vi "Periodic Tasks.vi"(8 "error in":errorcluster) -> ()   [LabVIEW 2014]
doc: "This VI runs in parallel to other tasks. It can contain as many user-defined periodic loops as you need. These can carry out PID or other sorts of timed response."
uses:
  <vilib>/Rock Robotics/WPI/Joystick/WPI_JoystickGetSetRefNum.vi
  <vilib>/Rock Robotics/WPI/RobotDrive/WPI_RobotDriveGetSetRefNum.vi
  Modules 2015/Desired Arm Position.vi
  Robot Global Data.vi
  <vilib>/Rock Robotics/Network Tables/SD Write Number.vi
panel:
  out "Voltage":dbl
  out "desired position":T1(graph)={"Desired Back Arm Position"=13.083464566929848, "Back Arm Distance (inches)"=14.0325}
  out "voltage 2":dbl
  out "Desired Back Arm Position":dbl
  in  "kd 2":dbl=0.01 format="%#_13g"
  in  "kp 2":dbl=0.15 format="%#_13g"
  out "voltage":dbl
  out "Desired Front Arm Position":dbl
  in  "kd":dbl=0.02 format="%#_13g"
  in  "kp":dbl=0.1 format="%#_13g"
  out "Front Arm Distance":dbl
  out "Back Arm Distance":dbl
  out "Angle":dbl
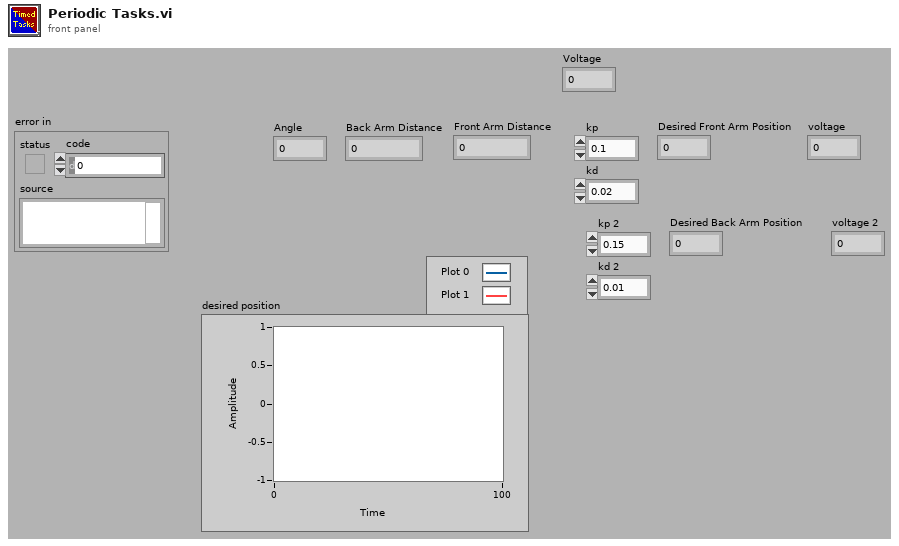
[diagram p1: front panel]
types:
  T1 = cluster{"Desired Back Arm Position":dbl, "Back Arm Distance (inches)":dbl}
  T2 = typedef "WPI_AnalogChannelDevRef.ctl" = cluster{"DevStatus":errorcluster, "Controller":T3, "Analog Channel":T4}
  T3 = typedef "FPGA_TypedefAnalogModule.ctl" = enum16{"Controller 1"}
  T4 = typedef "FPGA_AIChannel.ctl" = enum8{"AI 0", "AI 1", "AI 2", "AI 3", "AI MXP 0", "AI MXP 1", "AI MXP 2", "AI MXP 3", "Invalid"}
  T5 = typedef "WPI_DigitalInputDevRef.ctl" = cluster{"DevStatus":errorcluster, "DIO Channel":T6, "Controller":T7}
  T6 = typedef "FPGA_DIOChannel.ctl" = enum8{"DIO 0", "DIO 1", "DIO 2", "DIO 3", "DIO 4", "DIO 5", "DIO 6", "DIO 7", "DIO 8", "DIO 9", "DIO MXP 0", "DIO MXP 1", "DIO MXP 2", "DIO MXP 3", "DIO MXP 4", "DIO MXP 5", "DIO MXP 6", "DIO MXP 7", "DIO MXP 8", "DIO MXP 9", "DIO MXP 10", "DIO MXP 11", "DIO MXP 12", "DIO MXP 13", "DIO MXP 14", "DIO MXP 15", "Invalid"}
  T7 = typedef "FPGA_TypedefDigitalModule.ctl" = enum16{"Controller 1"}
  T8 = typedef "WPI_JoystickDevRef.ctl" = cluster{"Device":T9}
  T9 = typedef "WPI_JoystickDeviceEnum.ctl" = enum16{"USB 0", "USB 1", "USB 2", "USB 3", "USB 4", "USB 5"}
  T10 = typedef "WPI_RobotDriveDevRef.ctl" = cluster{"DevStatus":errorcluster, "Motors[]":T11[], "Square Inputs":bool, "Max Output":dbl}
  T11 = typedef "WPI_MotorControlDeviceRef.ctl" = cluster{"DeviceStatus":errorcluster, "Type":T12, "PWM":cluster{"Controller":T7, "PWM Channel":T13, "DeadBand":T14}, "CAN":cluster{"Device Number":u8, "Control Mode":T15, "Semaphore":T16, "Max Vout":dbl, "TalonSRX Control Mode":T17}, "Invert":bool, "TransformRef":T18, "InvTransformRef":T18}
  T12 = typedef "WPI_MotorControlType.ctl" = enum16{"PWM", "CAN", "CANTalonSRX"}
  T13 = typedef "FPGA_DIOPWMChannel.ctl" = enum8{"PWM 0", "PWM 1", "PWM 2", "PWM 3", "PWM 4", "PWM 5", "PWM 6", "PWM 7", "PWM 8", "PWM 9", "PWM MXP 0", "PWM MXP 1", "PWM MXP 2", "PWM MXP 3", "PWM MXP 4", "PWM MXP 5", "PWM MXP 6", "PWM MXP 7", "PWM MXP 8", "PWM MXP 9", "Invalid"}
  T14 = typedef "WPI_PWMDeadband.ctl" = cluster{"Name":string, "maxPositivePwm":i32, "minPositivePwm":i32, "centerPwm":i32, "maxNegativePwm":i32, "minNegativePwm":i32, "angularRange":u16}
  T15 = typedef "WPI_CANJaguar_ControlMode.ctl" = enum8{"Percent VBus", "Current", "Speed", "Position", "Voltage"}
  T16 = typedef "Semaphore RefNum" = refnum<k1>
  T17 = typedef "WPI_CANTalonSRX_APIControlMode.ctl" = enum8{"Percent VBus", "Speed", "Position", "Slave", "Unchanged / Invalid"}
  T18 = typedef "WPI_PWMTransform_ConPane.ctl" = refnum<vi>
  T19 = typedef "WPI_EncoderDevRef.ctl" = cluster{"DevStatus":errorcluster, "EncoderIndex":T20, "CounterIndex":T21, "DistancePerCount":dbl, "Decoding Type":T22}
  T20 = typedef "FPGA_EncoderIdx.ctl" = enum8{"Enc 0", "Enc 1", "Enc 2", "Enc 3", "Enc 4", "Enc 5", "Enc 6", "Enc 7", "Invalid"}
  T21 = typedef "FPGA_CounterCtrSystemIndex.ctl" = enum8{"Ctr 0", "Ctr 1", "Ctr 2", "Ctr 3", "Ctr 4", "Ctr 5", "Ctr 6", "Ctr 7", "Invalid"}
  T22 = typedef "WPI_EncoderType.ctl" = enum16{"1x", "2x", "4x"}
  T23 = cluster{"JoystickDevRef":T8, "RobotDriveDevRef":T10}
  T24 = typedef "WPI_GyroDevRef.ctl" = cluster{"DevStatus":errorcluster, "Analog Module":T3, "Analog Channel":T4, "Offset":dbl, "Gain (VoltsPerDegree/Second)":dbl}
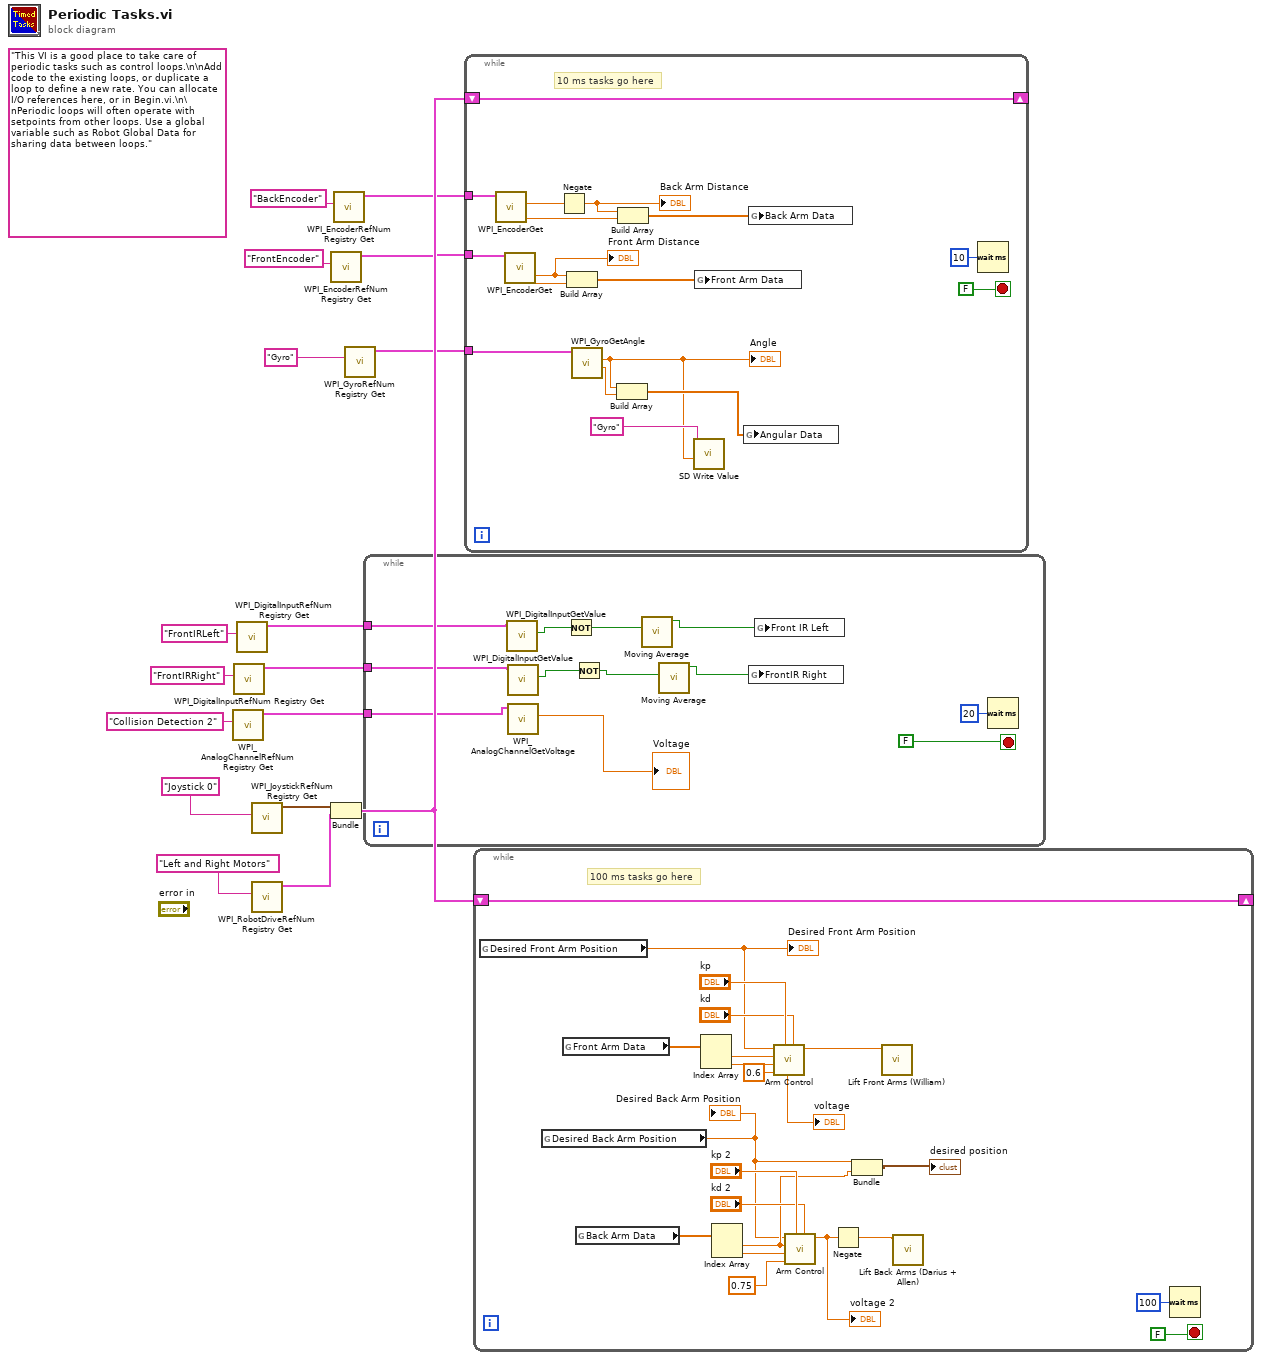
[diagram p0: block diagram]
diagram:
  (unwired) "This VI is a good place to take care of periodic tasks such as control loops.\n\nAdd code to the existing loops, or duplicate a loop to define a new rate. You can allocate I/O references here, or in Begin.vi.\n\nPeriodic loops will often operate with setpoints from other loops. Use a global variable such as Robot Global Data for sharing data between loops."
  n1 = call <vilib>:"WPI_AnalogChannelRefNum Registry Get.vi"("refnum name"="Collision Detection 2") -> ("AIDeviceRef"=w2:T2)  [unwired: 9 in, 1 out]
  n2 = call <vilib>:"WPI_DigitalInputRefNum Registry Get.vi"("refnum name"="FrontIRRight") -> ("DigitalInputDevRef"=w3:T5)  [unwired: 9 in, 1 out]
  n3 = call <vilib>:"WPI_DigitalInputRefNum Registry Get.vi"("refnum name"="FrontIRLeft") -> ("DigitalInputDevRef"=w4:T5)  [unwired: 9 in, 1 out]
  n4 = call <vilib>:"WPI_JoystickRefNum Registry Get.vi"("refnum name"="Joystick 0") -> ("JoystickDevRef"=w15:T8)  [unwired: 1 in, 9 out]
  n5 = call <vilib>:"WPI_RobotDriveRefNum Registry Get.vi"("refnum name"="Left and Right Motors") -> ("RobotDriveDevRef"=w14:T10)  [unwired: 1 in, 9 out]
  n6 = call <vilib>:"WPI_EncoderRefNum Registry Get.vi"("refnum name"="FrontEncoder") -> ("EncoderDevRef"=w5:T19)  [unwired: 9 in, 1 out]
  n7 = Bundle("JoystickDevRef"=w15, "RobotDriveDevRef"=w14) -> (w13:T23)  [unwired: 1 out]
  n8 = call <vilib>:"WPI_EncoderRefNum Registry Get.vi"("refnum name"="BackEncoder") -> ("EncoderDevRef"=w9:T19)  [unwired: 9 in, 1 out]
  n9 = call <vilib>:"WPI_GyroRefNum Registry Get.vi"("refnum name"="Gyro") -> ("GyroDevRef"=w12:T24)  [unwired: 9 in, 1 out]
  n10 = while {
    tunnel: w4 -> [w28]
    tunnel: w3 -> [w27]
    tunnel: w2 -> [w19]
    stop <- FALSE stop-if-true
    n11 = call <vilib>:"WPI_DigitalInputGetValue.vi"("DigitalInputDevRef"=w28) -> ("Value"=w25:bool)  [unwired: 8 in, 2 out]
    n12 = call <vilib>:"WPI_DigitalInputGetValue.vi"("DigitalInputDevRef"=w27) -> ("Value"=w24:bool)  [unwired: 8 in, 2 out]
    n13 = call <vilib>:"WPI_AnalogChannelGetVoltage.vi"("AIDeviceRef"=w19) -> ("Voltage"=→"Voltage":dbl)  [unwired: 8 in, 2 out]
    n14 = Not(x=w25) -> (.not. x?=w23:bool)
    n15 = Not(x=w24) -> (.not. x?=w21:bool)
    n16 = call "Moving Average.vi"("Value"=w23) -> ("Moving Boolean Average"=w22:bool)  [unwired: 10 in]
    n17 = call "Moving Average.vi"("Value"=w21) -> ("Moving Boolean Average"=w20:bool)  [unwired: 10 in]
    n18 = global write "Robot Global Data.vi" "FrontIR Right"(w20) -> ()
    n19 = global write "Robot Global Data.vi" "Front IR Left"(w22) -> ()
    n20 = Wait (ms)(milliseconds to wait=u32 20) -> ()  [unwired: 1 out]
  }
  n21 = while {
    shift-right: [w44] -> _
    shift-left: w13 -> [w44]
    tunnel: w12 -> [w43]
    tunnel: w9 -> [w42]
    tunnel: w5 -> [w40]
    stop <- FALSE stop-if-true
    # "10 ms tasks go here"
    n22 = call <vilib>:"WPI_EncoderGet.vi"("EncoderDevRef"=w42) -> ("Distance"=w31:dbl, "Rate"=w36:dbl)  [unwired: 5 in, 4 out]
    n23 = call <vilib>:"WPI_EncoderGet.vi"("EncoderDevRef"=w40) -> ("Distance"=w32:dbl, "Rate"=w34:dbl)  [unwired: 5 in, 4 out]
    "Front Arm Distance" <- w32
    n24 = Negate(x=w31) -> (-x=w30:dbl)
    "Back Arm Distance" <- w30
    n25 = Build Array(w32, w34) -> (w33:dbl[])
    n26 = call <vilib>:"WPI_GyroGetAngle.vi"("GyroDevRef"=w43) -> ("Angular Rate"=w39:dbl, "Angle"=w37:dbl)  [unwired: 7 in, 2 out]
    "Angle" <- w37
    n27 = Build Array(w37, w39) -> (w38:dbl[])
    n28 = Build Array(w30, w36) -> (w35:dbl[])
    n29 = call-poly <vilib>:"SD Write Value.vi"("Numeric"=w37, "Name"="Gyro") -> ()  [unwired: 8 in, 2 out]
    n30 = global write "Robot Global Data.vi" "Front Arm Data"(w33) -> ()
    n31 = global write "Robot Global Data.vi" "Angular Data"(w38) -> ()
    n32 = global write "Robot Global Data.vi" "Back Arm Data"(w35) -> ()
    n33 = Wait (ms)(milliseconds to wait=u32 10) -> ()  [unwired: 1 out]
  }
  n34 = while {
    shift-right: [w65] -> _
    shift-left: w13 -> [w65]
    stop <- FALSE stop-if-true
    # "100 ms tasks go here"
    n35 = global read "Desired Arm Position.vi" "Desired Front Arm Position"() -> (w47:dbl)
    "Desired Front Arm Position" <- w47
    n36 = global read "Desired Arm Position.vi" "Desired Back Arm Position"() -> (w49:dbl)
    "Desired Back Arm Position" <- w49
    n37 = global read "Robot Global Data.vi" "Front Arm Data"() -> (w64:dbl[])
    n38 = global read "Robot Global Data.vi" "Back Arm Data"() -> (w60:dbl[])
    n39 = Index Array(array=w64) -> (element #1=w52:dbl, element #2=w63:dbl)  [unwired: 2 in]
    n40 = Index Array(array=w60) -> (element #1=w51:dbl, element #2=w59:dbl)  [unwired: 2 in]
    n41 = call "Arm Control.vi"("kd"="kd", "kp"="kp", "Range"=0.6, "Current Speed"=w63, "Current Height"=w52, "Desired Height"=w47) -> ("Motor Output"=w53:dbl)  [unwired: 4 in, 1 out]
    "voltage" <- w53
    n42 = call "Arm Control.vi"("kd"="kd 2", "kp"="kp 2", "Range"=0.75, "Current Speed"=w59, "Current Height"=w51, "Desired Height"=w49) -> ("Motor Output"=w56:dbl)  [unwired: 4 in, 1 out]
    "voltage 2" <- w56
    n43 = Negate(x=w56) -> (-x=w55:dbl)
    n44 = Bundle("Desired Back Arm Position"=w49, "Back Arm Distance (inches)"=w51) -> (→"desired position":T1)  [unwired: 1 in]
    n45 = call "Lift Front Arms (William).vi"("Motor Output"=w53) -> ()  [unwired: 9 in, 2 out]
    n46 = call "Lift Back Arms (Darius + Allen).vi"("Motor Output"=w55) -> ()  [unwired: 9 in, 2 out]
    n47 = Wait (ms)(milliseconds to wait=u32 100) -> ()  [unwired: 1 out]
  }
